vi "Create All Message Queues.vi"(8 "error in (no error)":T1 caption="entrée d'erreur (pas d'erreur)", 11 "Stop Event":refnum<user-event>) -> (0 "error out":T1 caption="sortie d'erreur", 3 "Fifo":T2)   [LabVIEW 2020, in "Message Queue.lvlib"]
doc: "Ce VI crée et initialise toutes les files d'attente de messages de l'application. Si votre application requiert plusieurs files d'attente de messages, cliquez sur la constante \"Message Queues\" ci-dessus avec le bouton droit et sélectionnez Ouvrir la déf. de type. Ajoutez les nouvelles files d'attente de messages à la définition de type puis initialisez-les dans ce VI."
uses:
  Message Queue.lvlib
  All Message Queues.ctl
  Message Cluster.ctl
  Calculatrice/controls/ctrl_Ref.ctl
  Calculatrice/controls/ctrl_Event_Ref.ctl
  Calculatrice/controls/ctrl_UI_Ref.ctl
  Enqueue Message (Single).vi
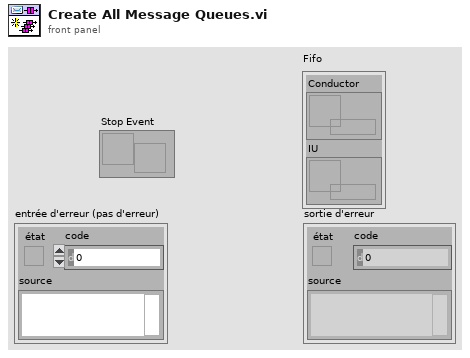
[diagram p1: front panel]
types:
  T1 = cluster{"état":bool, "code":i32, "source":string}
  T2 = typedef "Message Queue.lvlib/All Message Queues.ctl" = cluster{"Conductor":refnum<queue>, "IU":refnum<queue>}
  T3 = typedef "ctrl_Ref.ctl" = cluster{"Fifo":T2, "Event":T4, "UI":T5}
  T4 = typedef "ctrl_Event_Ref.ctl" = cluster{"Stop Event":refnum<user-event>}
  T5 = typedef "ctrl_UI_Ref.ctl" = cluster{"Display":refnum<vi>}
  T6 = cluster{"[0]":refnum<queue>, "[1]":refnum<queue>}
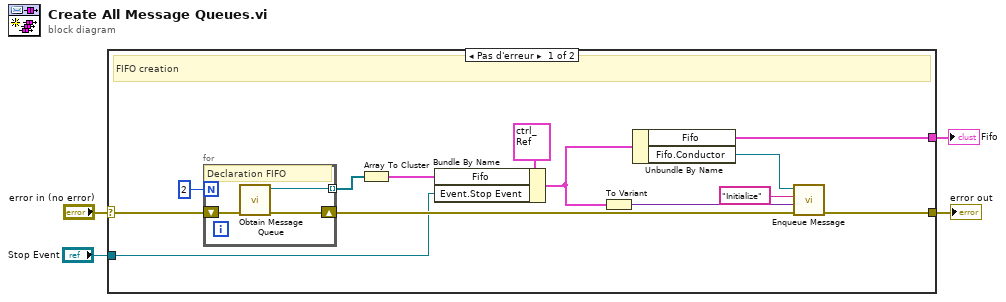
[diagram p0: block diagram]
diagram:
  n1 = case shown="Pas d'erreur" "error in (no error)" {
    selector: "error in (no error)" -> [w16 w21]
    tunnel: [w17 w21] -> w4
    tunnel: [w8 _] -> w3
    tunnel: "Stop Event" -> [w9 _]
    frame No Error {
      # "FIFO creation"
      n2 = for {
        N: 2 -> [_]
        tunnel: [w18] -> w12 mode=indexing
        shift-right: [w19] -> w15
        shift-left: w16 -> [w20]
        # "Declaration FIFO"
        n3 = call "Obtain Message Queue.vi"("error in (no error)"=w20) -> ("error out"=w19:T1, "File d'attente de messages"=w18:refnum<queue>)  [unwired: 9 in]
      }
      n4 = Array To Cluster(array=w12) -> (cluster=w10:T6)
      n5 = Bundle By Name(cluster=T3 {"Fifo"={"Conductor"=refnum, "IU"=refnum}, "Event"={"Stop Event"=refnum}, "UI"={"Display"=refnum}} ("Ref"), "Fifo"=w10, "Event.Stop Event"=w9) -> (w6:T3)
      n6 = To Variant(anything=w6) -> (Variant=w5:variant)
      n7 = Unbundle By Name(w6) -> ("Fifo"=w8:T2, "Fifo.Conductor"=w7:refnum<queue>)
      n8 = call-poly "Enqueue Message.vi"("error in (no error)"=w15, "Données de message"=w5, "Message"="Initialize", "File d'attente de messages"=w7) -> ("error out"=w17:T1)  [unwired: 6 in, 1 out]
    }
    frame Error {
    }
  }
  "Fifo" <- w3
  "error out" <- w4
